vi "Normal Moments.vi"(9 "std":dbl=1.0, 10 "mean":dbl, 11 "x":dbl) -> (0 "error":i32, 2 "variance":dbl=1.0, 3 "mean":dbl)   [LabVIEW 2014, in "NI_Gmath.lvlib"]
doc: "Returns the expected mean and variance of the random variate X, where X describes the selected distribution type. You must manually select the polymorphic instance to use."
uses:
  NI_Gmath.lvlib
  st_error_code.ctl
panel:
  # "Normal Moments"
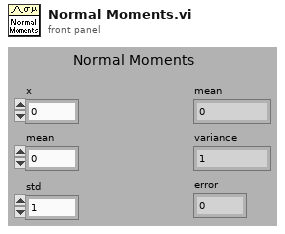
[diagram p1: front panel]
types:
  T1 = typedef "NI_Gmath.lvlib/st_error_code.ctl" = i32
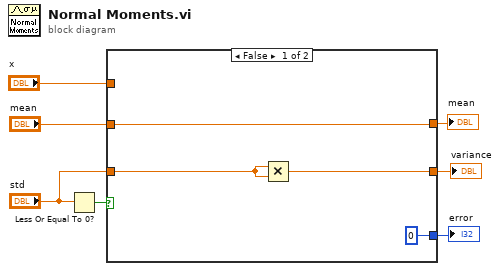
[diagram p0: block diagram]
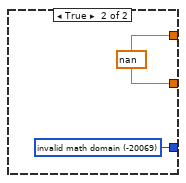
[diagram p2: hidden frame]
diagram:
  n1 = Less Or Equal To 0?(x="std") -> (x <= 0?=w7:bool)
  n2 = case shown="False" w7 {
    tunnel: "std" -> [w9 _]
    tunnel: [0 ("invalid math domain") w12] -> w5
    tunnel: [w10 w13] -> w4
    tunnel: "x" -> [_ _]
    tunnel: "mean" -> [w10 _]
    tunnel: [w8 w13] -> w1
    frame False {
      n3 = Multiply(x=w9, y=w9) -> (x*y=w8:dbl)
    }
    frame True {
      w12 = T1 -20069 items=["invalid math domain"=-20069, "Fourier interpolation size m >= n"=-20070, "empty array"=-20003] ("stat interp error code")
      w13 = nan
    }
  }
  "mean" <- w4
  "error" <- w5
  "variance" <- w1
